vi "connect.vi"(8 "error in (no error)":errorcluster, 11 "RabbitMQ Config":T1) -> (0 "error out":errorcluster, 3 "RabbitMQ Session Out":T2)   [LabVIEW 2019, in "rabbitmq.lvlib"]
uses:
  rabbitmq.lvlib
  session.ctl
  config.ctl
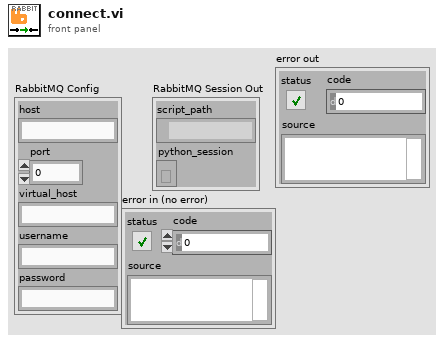
[diagram p1: front panel]
types:
  T1 = typedef "rabbitmq.lvlib/config.ctl" = cluster{"host":string, "port":i32, "virtual_host":string, "username":string, "password":string}
  T2 = typedef "rabbitmq.lvlib/session.ctl" = cluster{"script_path":path, "python_session":refnum<k35>}
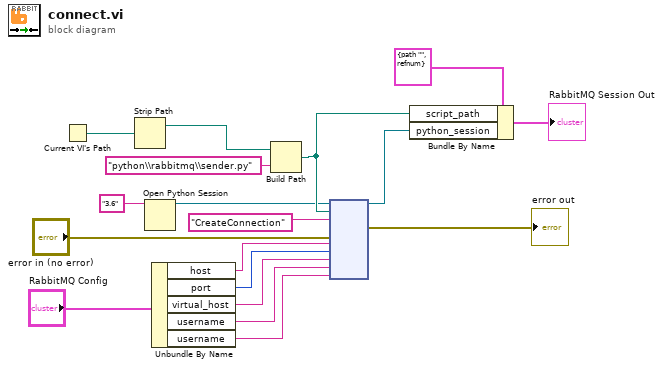
[diagram p0: block diagram]
diagram:
  n1 = Current VI's Path() -> (path=w2:path)
  n2 = Strip Path(path=w2) -> (stripped path=w1:path)  [unwired: 1 out]
  n3 = Open Python Session(python version="3.6" ("Python version")) -> (session out=w6:refnum<k35>)  [unwired: 2 in, 1 out]
  n4 = Unbundle By Name("RabbitMQ Config") -> ("host"=w10:string, "port"=w11:i32, "virtual_host"=w12:string, "username"=w13:string, "username"=w14:string)
  n5 = Build Path(base path=w1, name or relative path="python\\rabbitmq\\sender.py") -> (appended path=w18:path)
  n6 = node(w6, w18, "CreateConnection" ("function name"), "error in (no error)", w10, w11, w12, w13, w14) -> (w16:refnum<k35>, →"error out":errorcluster)  [unwired: 7 in, 2 out]
  n7 = Bundle By Name(cluster=T2 {"script_path"=path "", "python_session"=refnum}, "script_path"=w18, "python_session"=w16) -> (→"RabbitMQ Session Out":T2)
